vi "Configure Aperture.vi"(8 "error in (no error)":errorcluster, 9 "Averaging Factor (1)":i32=1, 10 "Measurement Time (1: Medium)":u16(ring)=1 items=["Short", "Medium", "Long"], 11 "VISA resource name":refnum<visa-resource-name>) -> (0 "error out":errorcluster, 3 "VISA resource name out":refnum<visa-resource-name>)   [LabVIEW 2019, in "Agilent E4980.lvlib"]
doc: "Sets the measurement time mode and the averaging factor."
uses:
  Agilent E4980.lvlib
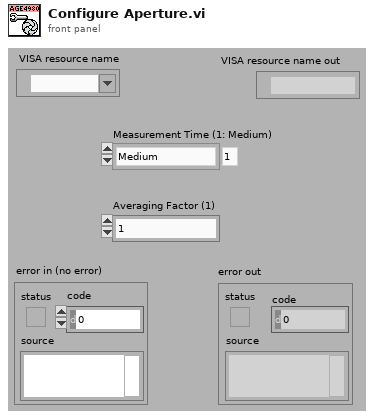
[diagram p1: front panel]
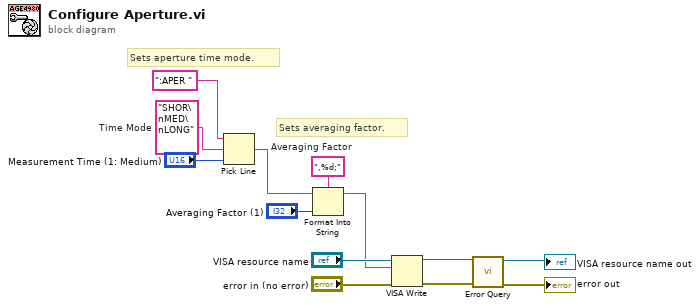
[diagram p0: block diagram]
diagram:
  w9 = ",%d;"  # Averaging Factor
  w12 = "SHOR\nMED\nLONG"  # Time Mode
  # "Sets aperture time mode."
  # "Sets averaging factor."
  n1 = Pick Line(string ("")=":APER ", multi-line string=w12, line index="Measurement Time (1: Medium)") -> (output string=w10:string)
  n2 = Format Into String(format string=w9, initial string=w10, "Averaging Factor (1)") -> (resulting string=w6:string)  [unwired: 1 in, 1 out]
  n3 = VISA Write(VISA resource name="VISA resource name", write buffer=w6, error in (no error)="error in (no error)") -> (VISA resource name out=w5:refnum<visa-resource-name>, error out=w4:errorcluster)  [unwired: 1 out]
  n4 = call "Error Query.vi"("error in (no error)"=w4, "VISA resource name"=w5) -> ("error out"=→"error out":errorcluster, "VISA resource name out"=→"VISA resource name out":refnum<visa-resource-name>)  [unwired: 6 in, 2 out]
